vi "Export_subVi.vi"(8 "error in (no error)":errorcluster, 11 "PMS_Data":T1) -> (0 "error out":errorcluster)   [LabVIEW 2019]
uses:
  Type Definitions/PMS_Data.ctl
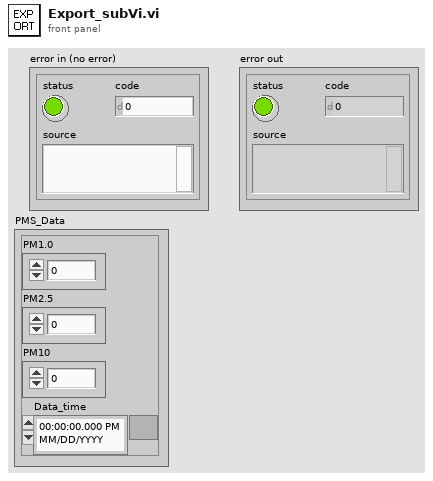
[diagram p1: front panel]
types:
  T1 = typedef "PMS_Data.ctl" = cluster{"PM1.0":i32, "PM2.5":i32, "PM10":i32, "Data_time":timestamp}
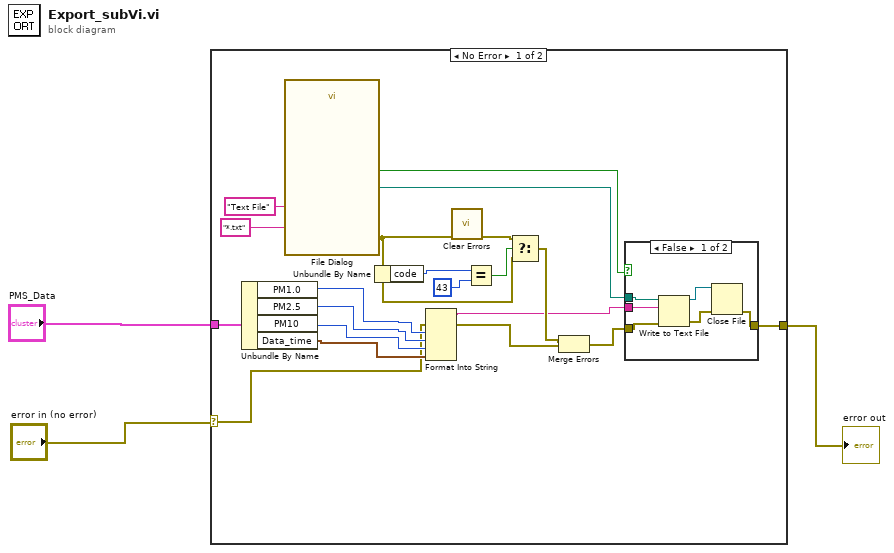
[diagram p0: block diagram]
diagram:
  n1 = case shown="No Error" "error in (no error)" {
    selector: "error in (no error)" -> [w6 w31]
    tunnel: [w21 w31] -> w3
    tunnel: "PMS_Data" -> [w11 _]
    frame No Error {
      n2 = Unbundle By Name(w11) -> ("PM1.0"=w10:i32, "PM2.5"=w9:i32, "PM10"=w8:i32, "Data_time"=w7:timestamp)
      n3 = call "File Dialog"("pattern (all files)"="*.txt", "pattern label"="Text File") -> ("selected path"=w19:path, "cancelled"=w20:bool, "error out"=w15:errorcluster)  [unwired: 10 in, 1 out]
      n4 = Unbundle By Name(w15) -> ("code"=w18:i32)
      n5 = Format Into String(error in=w6, w10, w9, w8, w7) -> (resulting string=w4:string, error out=w5:errorcluster)  [unwired: 2 in]
      n6 = call <vilib>:"Clear Errors.vi"("error in (no error)"=w15) -> ("error out"=w14:errorcluster)  [unwired: 5 in, 1 out]
      n7 = Equal?(x=w18, y=43) -> (x = y?=w16:bool)
      n8 = Select(t=w14, s=w16, f=w15) -> (s? t:f=w13:errorcluster)
      n9 = Merge Errors(w13, w5) -> (w12:errorcluster)
      n10 = case shown="False" w20 {
        tunnel: w12 -> [w27 w30]
        tunnel: [w24 w30] -> w21
        tunnel: w19 -> [w29 _]
        tunnel: w4 -> [w28 _]
        frame False {
          n11 = Write to Text File(file (use dialog)=w29, text=w28, error in=w27) -> (refnum out=w26:refnum<file>, error out=w25:errorcluster)  [unwired: 1 in, 1 out]
          n12 = Close File(refnum=w26, error in=w25) -> (error out=w24:errorcluster)  [unwired: 1 out]
        }
        frame True {
        }
      }
    }
    frame Error {
    }
  }
  "error out" <- w3
